vi "Do.vi"(8 "error in":errorcluster, 10 "Actor in":refnum<class "Actor.lvclass">, 11 "Configuration File Access Msg":refnum<class "Configuration Save Msg.lvclass">) -> (0 "error out":errorcluster, 2 "Actor out":refnum<class "Actor.lvclass">)   [LabVIEW 2018, in "EMS User Interface Actor.lvlib" / "Configuration Save Msg.lvclass"]
doc: "This VI delivers the message to the actor by calling the appropriate method(s) on the actor."
uses:
  Configuration Save Msg.lvclass
  C:/Users/Administrator/Desktop/2018LabVIEW EMS/Dialog Actors/File Dialog Actor/File Dialog Messages/Return File Path Msg/Return File Path Msg.lvclass
  <vilib>/ActorFramework/Actor/Actor.lvclass
  EMS User Interface/EMS User Interface.lvclass
  C:/Program Files (x86)/National Instruments/LabVIEW 2018/vi.lib/ActorFramework/Actor/Actor.lvclass
  C:/Users/Administrator/Desktop/2018LabVIEW EMS/EMS Generic Actor/EMS Generic/EMS Generic.lvclass
  EMS User Interface/Controls/Configuration/File Access Command.ctl
  Dialog Actors/File Dialog Actor/File Dialog Messages/Return File Path Msg/Return File Path Msg.lvclass/Return File Path Msg.ctl
  EMS Generic Actor/EMS Generic/EMS Generic.lvclass
  Dialog Actors/File Dialog Actor/File Dialog Messages/Return File Path Msg/Return File Path Msg.lvclass
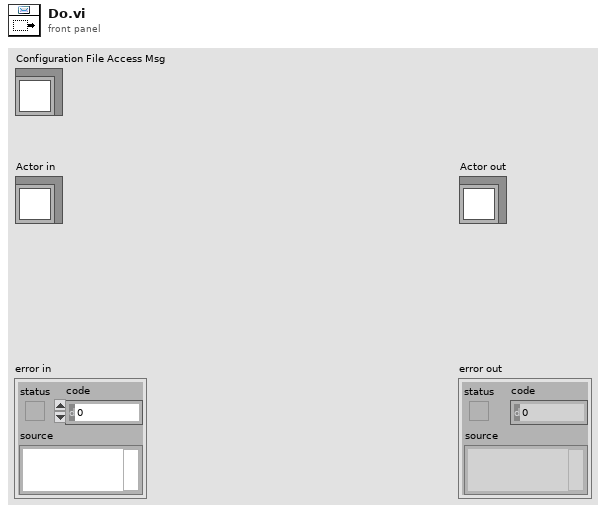
[diagram p1: front panel]
types:
  T1 = typedef "EMS User Interface Actor.lvlib/EMS User Interface.lvclass/File Access Command.ctl" = enum16{"Read", "Write"}
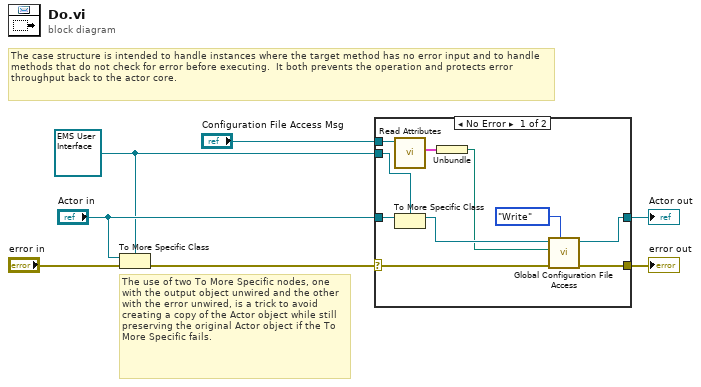
[diagram p0: block diagram]
diagram:
  w2 = refnum<class "EMS User Interface.lvclass"> refnum ("Actor in")
  # "The use of two To More Specific nodes, one with the output object unwired and the other with the error unwired, is a trick to avoid creating a copy of the Actor object while still preserving the original Actor object if the To More Specific fails."
  # "The case structure is intended to handle instances where the target method has no error input and to handle methods that do not check for error before executing.  It both prevents the operation and protects error throughput back to the actor core."
  n1 = To More Specific Class(target class=w2, reference="Actor in", error in="error in") -> (error out=w6:errorcluster)  [unwired: 1 out]
  n2 = case shown="No Error" w6 {
    selector: w6 -> [w15 w19]
    tunnel: [w17 w19] -> w5
    tunnel: [w16 w18] -> w4
    tunnel: "Actor in" -> [w14 w18]
    tunnel: w2 -> [w13 _]
    tunnel: "Configuration File Access Msg" -> [w10 _]
    frame No Error {
      n3 = call "Read Attributes.vi"("Return File Path Msg"=w10) -> ("Payload"=w11:cluster{"File Path":path})  [unwired: 10 in]
      n4 = To More Specific Class(target class=w13, reference=w14) -> (specific class reference=w12:refnum<class "EMS User Interface.lvclass">)  [unwired: 1 in, 1 out]
      n5 = Unbundle(w11) -> ("File Path"=w9:path)
      n6 = call "Global Configuration File Access.vi"("Command"=File_Access_Command."Write", "error in"=w15, "configuration file path"=w9, "EMS Generic in"=w12) -> ("error out"=w17:errorcluster, "EMS Generic out"=w16:refnum<class "EMS User Interface.lvclass">)  [unwired: 6 in]
    }
    frame Error {
      # "If type check fails, pass the original object out again."
    }
  }
  "error out" <- w5
  "Actor out" <- w4
